vi "Write Log Message.vi"(8 "error in (no error)":errorcluster, 10 "Message":string, 11 "Model in":refnum<class "Model.lvclass">) -> (0 "error out":errorcluster, 3 "Model out":refnum<class "Model.lvclass">)   [LabVIEW 2016, in "Model.lvclass"]
uses:
  Model.lvclass
  Model.lvclass/Model.ctl
  Test Log/Test Log/OperationsLog.lvclass
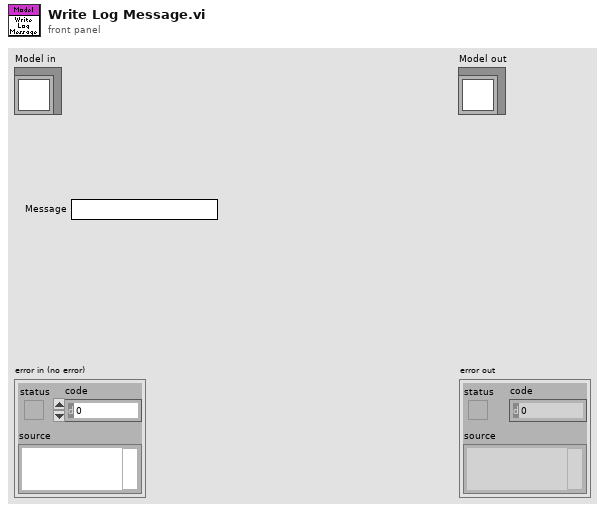
[diagram p1: front panel]
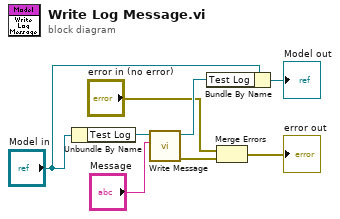
[diagram p0: block diagram]
diagram:
  n1 = Unbundle By Name("Model in") -> ("Test Log"=w8:refnum<class "OperationsLog.lvclass">)
  n2 = call-dynamic "Write Message.vi"("Message"="Message", "Test Log in"=w8) -> ("error out"=w3:errorcluster, "Test Log out"=w5:refnum<class "OperationsLog.lvclass">)  [unwired: 8 in]
  n3 = Bundle By Name(cluster="Model in", "Test Log"=w5) -> (→"Model out":refnum<class "Model.lvclass">)
  n4 = Merge Errors("error in (no error)", w3) -> (→"error out":errorcluster)
